vi "Publish Updates.vi"(8 "error in (no error)":errorcluster, 11 "Timer in":refnum<class "Timer.lvclass">) -> (0 "error out":errorcluster, 3 "Timer out":refnum<class "Timer.lvclass">)   [LabVIEW 2024, in "Timer.lvlib" / "Timer.lvclass"]
uses:
  Timer.lvclass
  Timer.lvclass/Timer.ctl
  <vilib>/ActorFramework/Actor/Actor.lvclass
  Controller/Controller Messages/Timer Update Display Msg/Timer Update Display Msg.lvclass
  Applications/National Instruments/LabVIEW 2024 64-bit/vi.lib/ActorFramework/Actor/Actor.lvclass
  Users/elijahkerry/challenge-of-champions/Timer/Timer/Timer.lvclass
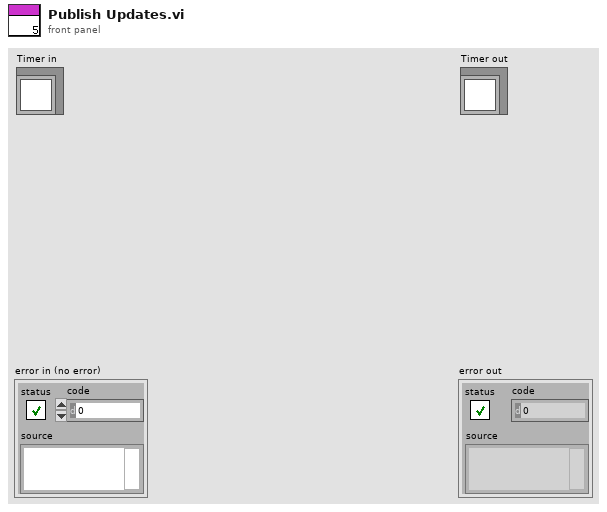
[diagram p1: front panel]
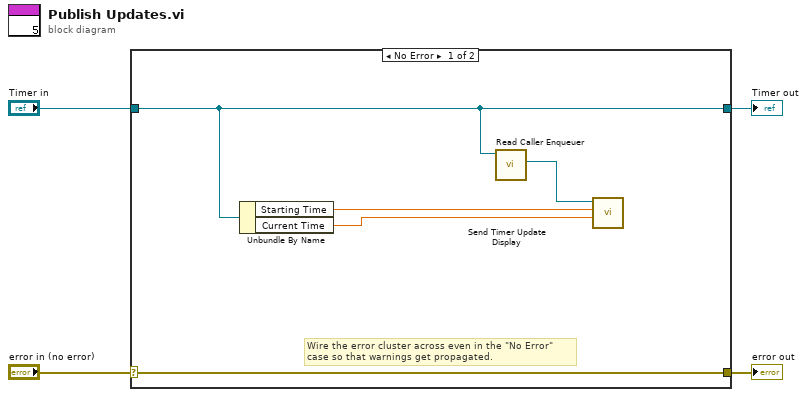
[diagram p0: block diagram]
diagram:
  n1 = case shown="No Error" "error in (no error)" {
    selector: "error in (no error)" -> [w9 w11]
    tunnel: [w9 w11] -> w3
    tunnel: [w7 w10] -> w1
    tunnel: "Timer in" -> [w7 w10]
    frame No Error {
      # "Wire the error cluster across even in the \"No Error\"\ncase so that warnings get propagated."
      n2 = Unbundle By Name(w7) -> ("Starting Time"=w6:dbl, "Current Time"=w5:dbl)
      n3 = call <vilib>:"Read Caller Enqueuer.vi"("Actor"=w7) -> ("Caller Enqueuer"=w8:refnum<class "Message Enqueuer.lvclass">)  [unwired: 10 in]
      n4 = call "Send Timer Update Display.vi"("Current Time"=w5, "Starting Time"=w6, "Message Enqueuer"=w8) -> ()  [unwired: 7 in, 2 out]
    }
    frame Error {
    }
  }
  "error out" <- w3
  "Timer out" <- w1
